vi "Main.vi"() -> ()   [LabVIEW 2015]
doc: "The myRIO Project template acquires acceleration data from the onboard accelerometer and displays the changes of acceleration values in a waveform chart."
uses:
  <vilib>/myRIO/Common/Instrument Driver Framework/myRIO v1.0/Encoder/typedefs/Encoder Signal Mode.ctl
  <vilib>/myRIO/Instrument Drivers/Onboard IO/Encoder/typedefs/Encoder Reference.ctl
  <vilib>/myRIO/Common/Instrument Driver Framework/Utilities/typedefs/myRIO Generic Hardware Reference.ctl
  <vilib>/myRIO/Common/Instrument Driver Framework/Utilities/typedefs/Hardware Version Enum.ctl
  <vilib>/myRIO/Common/Instrument Driver Framework/Utilities/typedefs/myRIO v1.0 Reference.ctl
  <vilib>/myRIO/Common/Instrument Driver Framework/Utilities/typedefs/Generic FPGA Reference.ctl
  <vilib>/myRIO/Common/Instrument Driver Framework/myRIO v1.0/Encoder/typedefs/Encoder Channels Enum.ctl
  <vilib>/myRIO/Common/Instrument Driver Framework/myRIO v1.0/Encoder/typedefs/Encoder Configuration v1.0.ctl
  <vilib>/userdefined/High Color/nirio_resource_hc.ctl
  <vilib>/myRIO/Instrument Drivers/Onboard IO/PWM/typedefs/PWM Reference.ctl
  <vilib>/myRIO/Common/Instrument Driver Framework/myRIO v1.0/PWM/typedefs/PWM Channels Enum.ctl
  <vilib>/myRIO/Instrument Drivers/Onboard IO/PWM/typedefs/PWM Configuration.ctl
  <vilib>/myRIO/Common/Instrument Driver Framework/Utilities/vis/Is FPGA Ref Available.vi
  <vilib>/myRIO/Common/Instrument Driver Framework/myRIO v1.0/Encoder/vis/myRIO v1.1 Open Encoder.vi
  <vilib>/myRIO/Instrument Drivers/Onboard IO/Encoder/vis/Read.vi
  <vilib>/myRIO/Common/Instrument Driver Framework/myRIO v1.0/PWM/vis/myRIO v1.1 Open PWM.vi
  <vilib>/myRIO/Instrument Drivers/Onboard IO/PWM/vis/Set Duty Cycle and Frequency.vi
  <vilib>/myRIO/Common/Instrument Driver Framework/Utilities/vis/Validate Channels.vi
  <vilib>/myRIO/Common/Instrument Driver Framework/myRIO v1.0/Encoder/vis/myRIO v1.0 Reserve Encoder.vi
  <vilib>/myRIO/Common/Instrument Driver Framework/myRIO v1.0/PWM/vis/myRIO v1.0 Reserve PWM.vi
  <vilib>/myRIO/Common/Instrument Driver Framework/myRIO v1.0/UART/vis/myRIO v1.0 Close UART.vi
  <vilib>/myRIO/Common/Instrument Driver Framework/myRIO v1.0/Encoder/vis/myRIO v1.0 Build MUX Configuration Encoder.vi
  <vilib>/myRIO/Common/Instrument Driver Framework/myRIO v1.0/Resource Manager/vis/myRIO v1.0 Reserve Channel List.vi
  <vilib>/myRIO/Common/Instrument Driver Framework/myRIO v1.0/PWM/vis/myRIO v1.0 Build MUX Configuration PWM.vi
  <vilib>/myRIO/Common/Instrument Driver Framework/myRIO v1.0/Resource Manager/vis/myRIO v1.0 Create Configuration List.vi
  <vilib>/myRIO/Common/Instrument Driver Framework/myRIO v1.0/Resource Manager/vis/myRIO v1.0 Reserve Channel.vi
  <vilib>/myRIO/Common/Instrument Driver Framework/myRIO v1.0/Resource Manager/vis/myRIO v1.0 Unreserve Channel.vi
  <vilib>/myRIO/Common/Instrument Driver Framework/myRIO v1.0/Resource Manager/vis/myRIO v1.0 Build Mutex Name.vi
  <vilib>/Utility/VariantDataType/GetNumericInfo.vi
  <vilib>/Utility/error.llb/Error Cluster From Error Code.vi
  <vilib>/myRIO/Common/Instrument Driver Framework/myRIO v1.0/myRIO v1.1 Open.vi
  <vilib>/myRIO/Common/Instrument Driver Framework/Utilities/vis/IO Manager.vi
  <vilib>/myRIO/Common/Instrument Driver Framework/Utilities/vis/Configuration Manager.vi
  <vilib>/myRIO/Common/Instrument Driver Framework/myRIO v1.0/Resource Manager/vis/myRIO v1.0 Configure IO.vi
  <vilib>/myRIO/Common/Instrument Driver Framework/myRIO v1.0/myRIO v1.0 Close.vi
  <vilib>/myRIO/Common/Instrument Driver Framework/myRIO v1.0/Encoder/vis/myRIO v1.0 Configure Encoder.vi
  <vilib>/myRIO/Common/Instrument Driver Framework/myRIO v1.0/Encoder/vis/myRIO v1.0 Read Encoder.vi
  <vilib>/myRIO/Common/Instrument Driver Framework/myRIO v1.0/PWM/vis/myRIO v1.0 Write PWM.vi
  <vilib>/myRIO/Common/Instrument Driver Framework/Utilities/vis/FPGA Ref Manager.vi
  <vilib>/myRIO/Common/Instrument Driver Framework/myRIO v1.0/myRIO v1.0 Reset FPGA.vi
  <vilib>/myRIO/Common/Instrument Driver Framework/myRIO v1.0/IRQ/vis/myRIO v1.0 IRQ Info FGV.vi
  <vilib>/myRIO/Common/Instrument Driver Framework/myRIO v1.0/IRQ/vis/myRIO v1.0 Timer IRQ Info FGV.vi
  <vilib>/myRIO/Common/Instrument Driver Framework/myRIO v1.0/IRQ/vis/myRIO v1.0 ISR Agent.vi
  <vilib>/myRIO/Express VI/Onboard IO/Encoder/Encoder Express VI.xnode
  <vilib>/myRIO/Common/Instrument Driver Framework/myRIO v1.0/Encoder/typedefs/Encoder Count Direction Enum.ctl
  <vilib>/myRIO/Instrument Drivers/Onboard IO/Encoder/vis/myRIO Encoder Open.xnode
  <vilib>/myRIO/Express VI/Onboard IO/PWM/PWM Express VI.xnode
  <vilib>/myRIO/Instrument Drivers/Onboard IO/PWM/vis/myRIO PWM Open.xnode
  <vilib>/myRIO/Instrument Drivers/Utilities/Utilities.lvlib
  <vilib>/myRIO/Instrument Drivers/Onboard IO/Encoder/Encoder.lvlib
  <vilib>/myRIO/Instrument Drivers/Onboard IO/PWM/PWM.lvlib
panel:
  out "Waveform Chart 2":dbl(graph)
  out "filtTheta":dbl
  in  "Boolean":bool
  out "Theta control 2":dbl
  out "Waveform Chart":dbl(graph)
  out "Theta control":dbl
  out "Control":bool
  out "dPhi":dbl(graph)
  out "dTheta":dbl(graph)
  in  "Swing up gain":dbl
  out "Rad dTheta":dbl
  out "Rad dPhi":dbl
  out "Rad Theta":dbl
  out "Rad Phi":dbl
  out "Direction Pend":dbl
  out "Counter Pend":dbl
  out "Direction Motor":dbl
  out "Counter Motor":dbl
  in  "Stop Button":bool
  out "error out":errorcluster
  # "Overview: The myRIO Project template acquires acceleration data from the onboard accelerometer and displays the changes of acceleration values in a waveform chart.\nInstructions:\n1. Check the myRIO target IP address in the project and make sure the target IP address is correct. \n2. Run this VI."
types:
  T1 = typedef "PWM.lvlib/PWM Reference.ctl" = cluster{"myRIO Reference":T2, "PWM Channels Enum":T6, "PWM Configuration":T7}
  T2 = typedef "myRIO Generic Hardware Reference.ctl" = cluster{"myRIO Model":T3, "myRIO Hardware Reference":T4}
  T3 = typedef "Hardware Version Enum.ctl" = enum16{"Unknown", "myRIO-1900", "myRIO-1950", "roboRIO"}
  T4 = typedef "myRIO v1.0 Reference.ctl" = cluster{"Generic FPGA Reference":T5, "Allow multiple opens":bool}
  T5 = typedef "Generic FPGA Reference.ctl" = refnum<k20>
  T6 = typedef "PWM Channels Enum.ctl" = enum16{"Not Connected", "C/PWM0", "C/PWM1", "A/PWM0", "A/PWM1", "A/PWM2", "B/PWM0", "B/PWM1", "B/PWM2", "PWM/PWM0", "PWM/PWM1", "PWM/PWM2", "PWM/PWM3", "PWM/PWM4", "PWM/PWM5", "PWM/PWM6", "PWM/PWM7", "PWM/PWM8", "PWM/PWM9"}
  T7 = typedef "PWM.lvlib/PWM Configuration.ctl" = cluster{"Frequency":dbl, "Duty Cycle":dbl}
  T8 = typedef "nirio_resource_hc.ctl" = tag
  T9 = typedef "Encoder.lvlib/Encoder Reference.ctl" = cluster{"myRIO Reference":T2, "Encoder Channels Enum":T10}
  T10 = typedef "Encoder Channels Enum.ctl" = enum16{"Not Connected", "C/ENC0", "C/ENC1", "A/ENC", "B/ENC", "DIO/ENC0", "DIO/ENC1", "DIO/ENC2", "DIO/ENC3", "DIO/ENC4"}
  T11 = typedef "Encoder Signal Mode.ctl" = enum16{"Quadrature phase signal", "Step and direction signal"}
  T12 = typedef "Encoder Count Direction Enum.ctl" = enum16{"Counting Up", "Counting Down"}
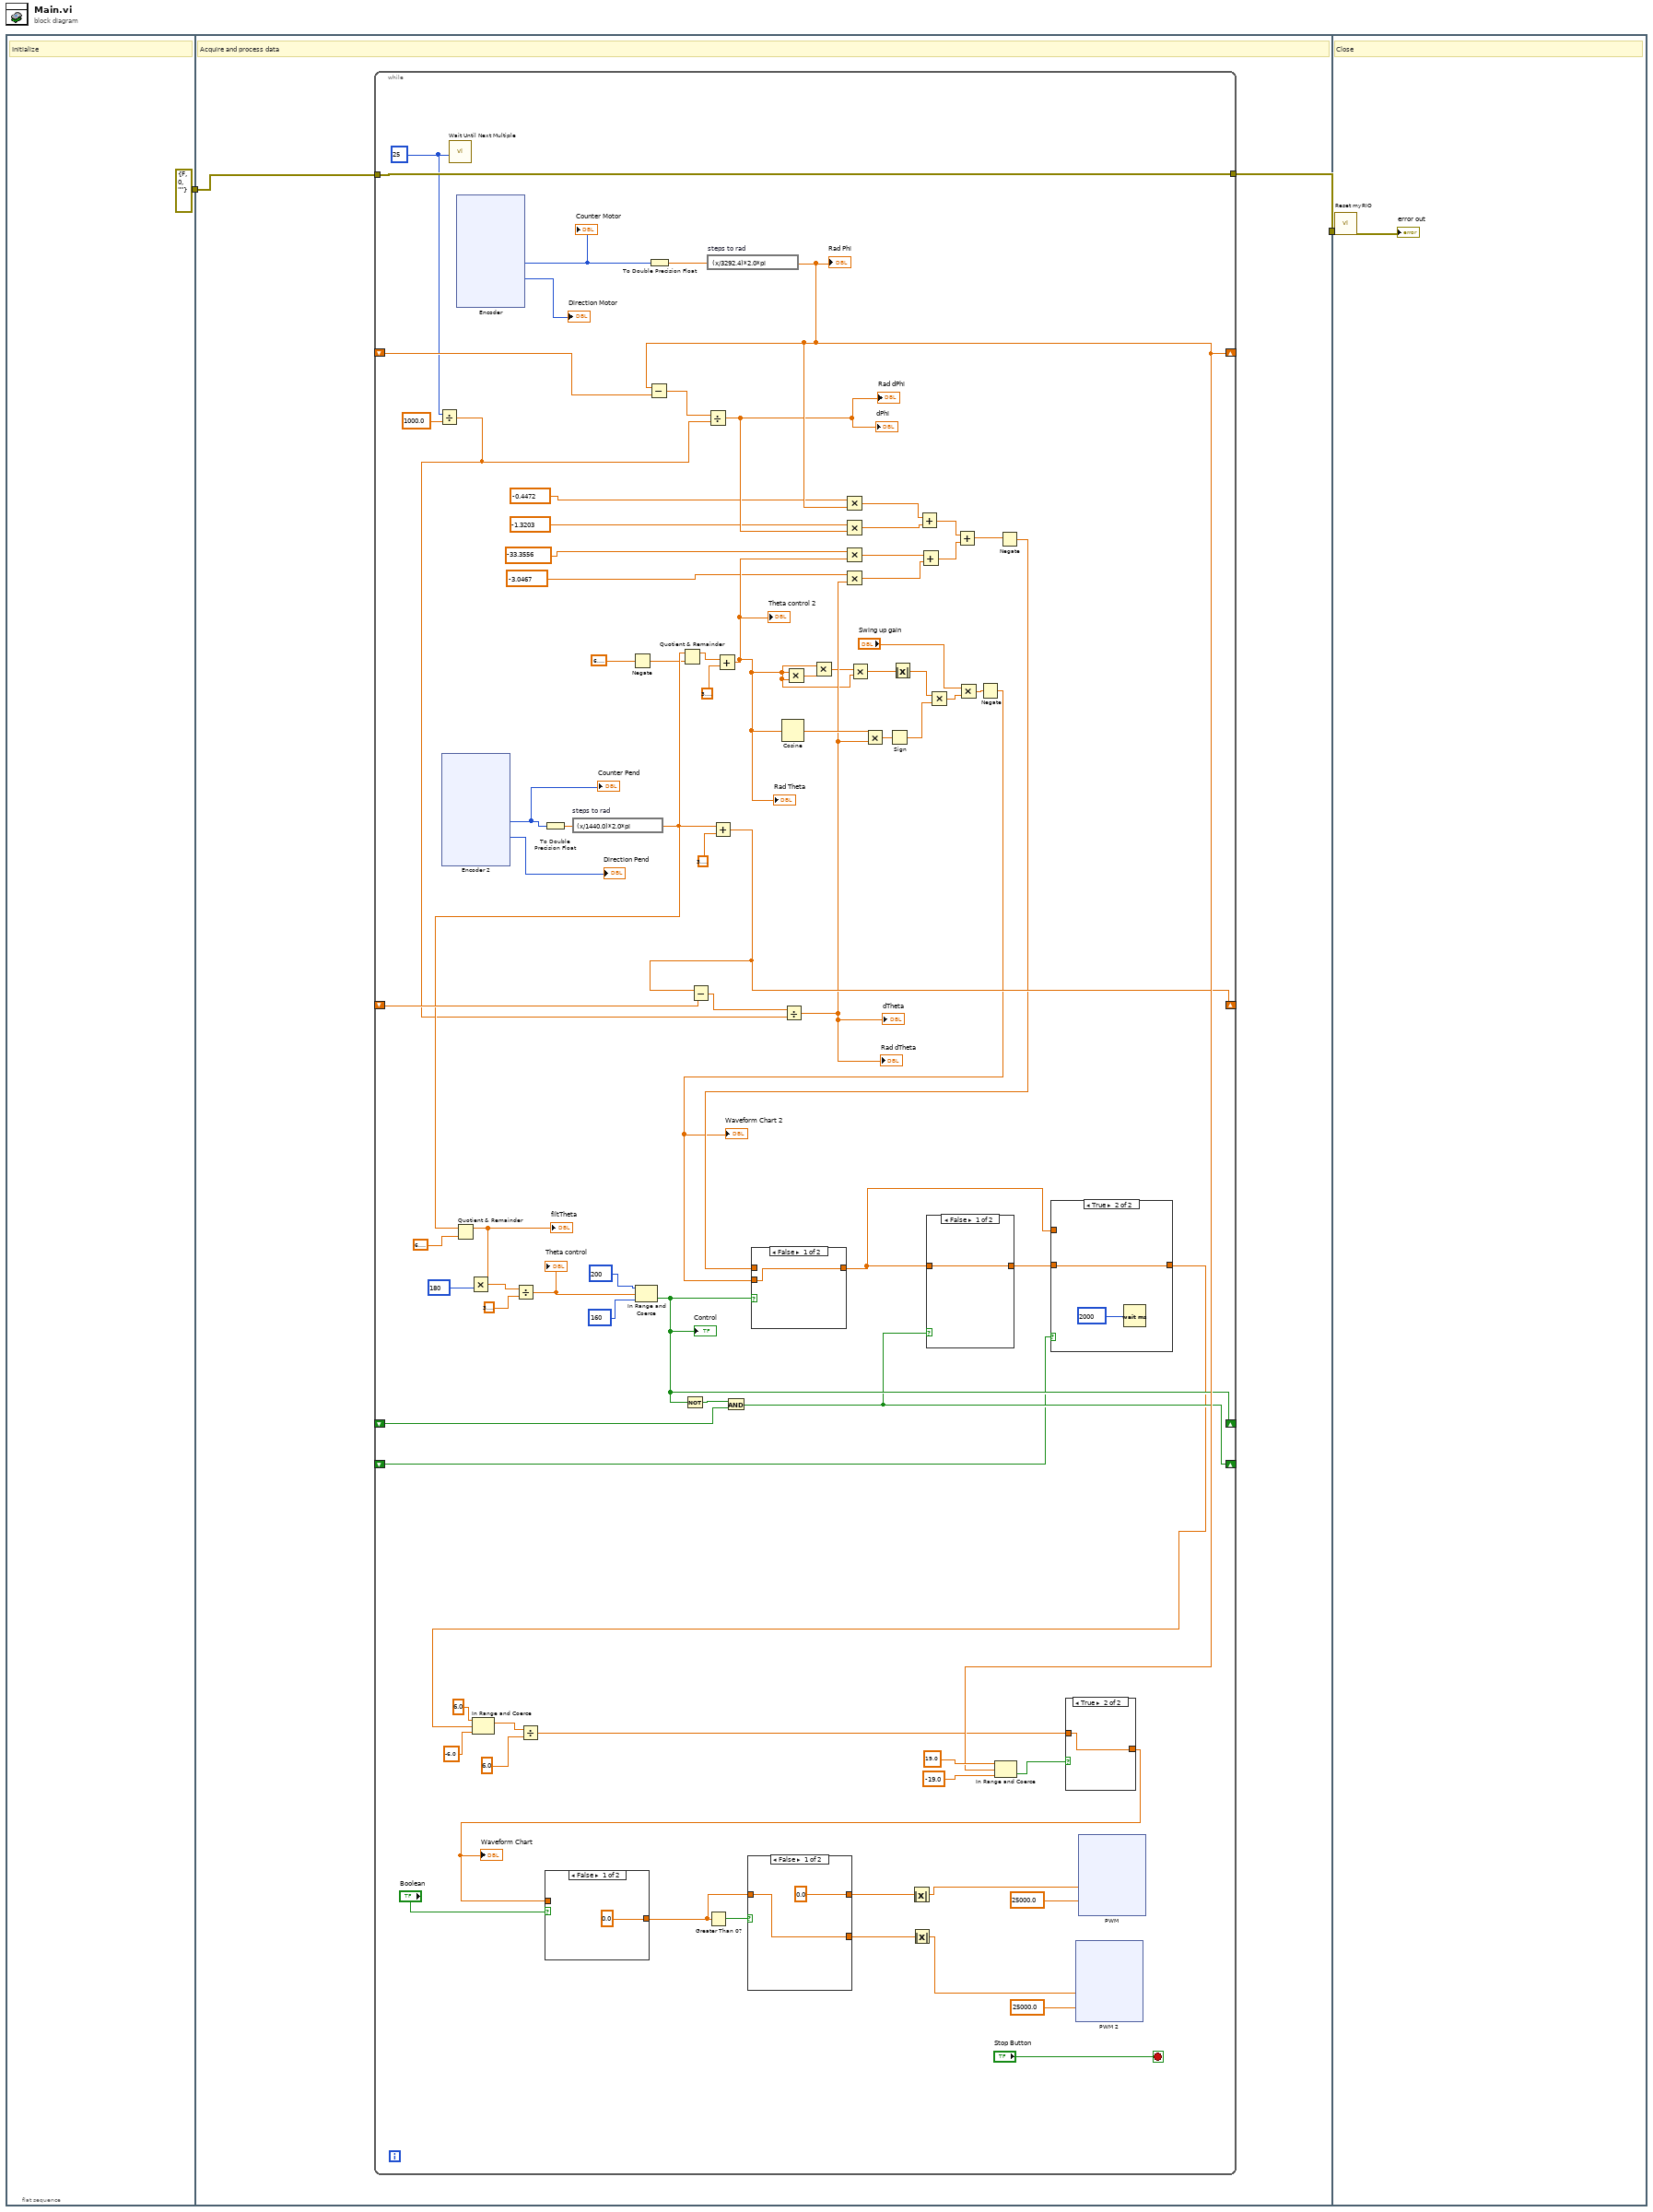
[diagram p0: block diagram]
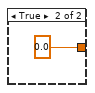
[diagram p3: hidden frame]
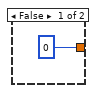
[diagram p6: hidden frame]
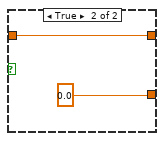
[diagram p7: hidden frame]
diagram:
  n1 = flat-sequence {
    tunnel: [errorcluster {"status"=FALSE, "code"=0, "source"=""} ("error in (no error)")] -> w2
    tunnel: w2 -> [w5]
    tunnel: [w4] -> w1
    tunnel: w1 -> [w267]
    frame #0 {
      # "Initialize"
    }
    frame #1 {
      # "Acquire and process data"
      n2 = while {
        tunnel: w5 -> [w78]
        tunnel: [w78] -> w4
        shift-right: [w60] -> _
        shift-left: _ -> [w77]
        shift-right: [w58] -> _
        shift-left: _ -> [w74]
        shift-right: [w13] -> _
        shift-left: _ -> [w12]
        shift-right: [w11] -> _
        shift-left: _ -> [w10]
        stop <- "Stop Button" stop-if-true
        w16 = u32 25 ("Count(mSec)")
        n3 = Divide(x=w16, y=1000.0) -> (x/y=w15:dbl)
        n4 = xnode "Encoder 2"() -> ("Counter Value"=w18:i32, "Counter Direction"=→"Direction Pend":enum16{"Counting Up", "Counting Down"})  [unwired: 2 in, 2 out]
        "Counter Pend" <- w18
        n5 = call "Wait Until Next Multiple"("Count(mSec)"=w16) -> ()  [unwired: 1 out]
        n6 = xnode "Encoder"() -> ("Counter Value"=w86:i32, "Counter Direction"=→"Direction Motor":T12)  [unwired: 2 in, 2 out]
        "Counter Motor" <- w86
        n7 = To Double Precision Float(number=w18) -> (double precision float=w85:dbl)
        n8 = expression code="(x/1440.0)*2.0*pi" "steps to rad"(w85) -> (w33:dbl)
        n9 = Quotient & Remainder(x=w33, y=6.283185307179586) -> (x-y*floor(x/y)=w49:dbl)  [unwired: 1 out]
        "filtTheta" <- w49
        n10 = Multiply(x=w49, y=180) -> (x*y=w47:dbl)
        n11 = Divide(x=w47, y=3.141592653589793) -> (x/y=w45:dbl)
        "Theta control" <- w45
        n12 = Negate(x=6.283185307179586) -> (-x=w30:dbl)
        n13 = In Range and Coerce(upper limit=200, x=w45, lower limit=160) -> (In Range?=w13:bool)  [unwired: 1 out]
        "Control" <- w13
        n14 = To Double Precision Float(number=w86) -> (double precision float=w84:dbl)
        n15 = Quotient & Remainder(x=w33, y=w30) -> (x-y*floor(x/y)=w31:dbl)  [unwired: 1 out]
        n16 = Not(x=w13) -> (.not. x?=w14:bool)
        n17 = expression code="(x/3292.4)*2.0*pi" "steps to rad"(w84) -> (w60:dbl)
        "Rad Phi" <- w60
        n18 = Subtract(x=w60, y=w77) -> (x-y=w76:dbl)
        n19 = Divide(x=w76, y=w15) -> (x/y=w59:dbl)
        "Rad dPhi" <- w59
        "dPhi" <- w59
        n20 = Add(x=w33, y=3.141592653589793) -> (x+y=w58:dbl)
        n21 = Subtract(x=w58, y=w74) -> (x-y=w75:dbl)
        n22 = Add(x=w31, y=3.141592653589793) -> (x+y=w28:dbl)
        "Rad Theta" <- w28
        "Theta control 2" <- w28
        n23 = And(x=w14, y=w12) -> (x .and. y?=w11:bool)
        n24 = Cosine(x=w28) -> (cos(x)=w72:dbl)
        n25 = Divide(x=w75, y=w15) -> (x/y=w57:dbl)
        "Rad dTheta" <- w57
        "dTheta" <- w57
        n26 = Multiply(x=w28, y=w28) -> (x*y=w64:dbl)
        n27 = Multiply(x=w28, y=w64) -> (x*y=w29:dbl)
        n28 = Multiply(x=-0.4472 ("element"), y=w60) -> (x*y=w51:dbl)
        n29 = Multiply(x=-1.3203 ("element"), y=w59) -> (x*y=w52:dbl)
        n30 = Multiply(x=-33.3556 ("element"), y=w28) -> (x*y=w53:dbl)
        n31 = Multiply(x=-3.0467 ("element"), y=w57) -> (x*y=w54:dbl)
        n32 = Multiply(x=w29, y=w28) -> (x*y=w27:dbl)
        n33 = Multiply(x=w72, y=w57) -> (x*y=w71:dbl)
        n34 = Sign(1:w71) -> (0:w73:dbl)
        n35 = Absolute Value(x=w27) -> (abs(x)=w65:dbl)
        n36 = Add(x=w51, y=w52) -> (x+y=w56:dbl)
        n37 = Add(x=w53, y=w54) -> (x+y=w55:dbl)
        n38 = Multiply(x=w65, y=w73) -> (x*y=w63:dbl)
        n39 = Add(x=w56, y=w55) -> (x+y=w42:dbl)
        n40 = Multiply(x="Swing up gain", y=w63) -> (x*y=w50:dbl)
        n41 = Negate(x=w50) -> (-x=w6:dbl)
        "Waveform Chart 2" <- w6
        n42 = In Range and Coerce(upper limit=19.0, x=w60, lower limit=-19.0 ("upper limit")) -> (In Range?=w66:bool)  [unwired: 1 out]
        n43 = Negate(x=w42) -> (-x=w37:dbl)
        n44 = case shown="False" w13 {
          tunnel: w37 -> [_ w97]
          tunnel: w6 -> [w96 _]
          tunnel: [w96 w97] -> w7
          frame False {
          }
          frame True {
          }
        }
        n45 = case shown="False" w11 {
          tunnel: w7 -> [w92 _]
          tunnel: [w92 0.0] -> w9
          frame False {
          }
          frame True {
          }
        }
        n46 = case shown="True" w10 {
          tunnel: w9 -> [_ w90]
          tunnel: [w89 w90] -> w8
          tunnel: w7 -> [w89 _]
          frame False {
          }
          frame True {
            n47 = Wait (ms)(milliseconds to wait=u32 2000) -> ()  [unwired: 1 out]
          }
        }
        n48 = In Range and Coerce(upper limit=6.0, x=w8, lower limit=-6.0) -> (coerced(x)=w38:dbl)  [unwired: 1 out]
        n49 = Divide(x=w38, y=6.0) -> (x/y=w24:dbl)
        n50 = case shown="True" w66 {
          tunnel: [0 w99] -> w23
          tunnel: w24 -> [_ w99]
          frame False {
          }
          frame True {
          }
        }
        "Waveform Chart" <- w23
        n51 = case shown="False" "Boolean" {
          tunnel: [0.0 ("upper limit") w95] -> w26
          tunnel: w23 -> [_ w95]
          frame False {
          }
          frame True {
          }
        }
        n52 = Greater Than 0?(x=w26) -> (x > 0?=w81:bool)
        n53 = case shown="False" w81 {
          tunnel: w26 -> [w101 w102]
          tunnel: [w101 0.0] -> w80
          tunnel: [0.0 w102] -> w79
          frame False {
          }
          frame True {
          }
        }
        n54 = Absolute Value(x=w79) -> (abs(x)=w36:dbl)
        n55 = Absolute Value(x=w80) -> (abs(x)=w35:dbl)
        n56 = xnode "PWM 2"("Duty Cycle"=w35, "Frequency [Hz]"=25000.0) -> ()  [unwired: 1 in, 1 out]
        n57 = xnode "PWM"("Duty Cycle"=w36, "Frequency [Hz]"=25000.0) -> ()  [unwired: 1 in, 1 out]
      }
    }
    frame #2 {
      # "Close"
      n58 = call <vilib>:"Reset myRIO.vi"("error in (no error)"=w267) -> ("error out"=→"error out":errorcluster)  [unwired: 10 in]
    }
  }
